vi "StopSong.vi"(8 "error in (no error)":errorcluster, 10 "Message Queues in":T1, 11 "UI Refs in":T2) -> (0 "error out":errorcluster, 2 "Message Queues out":T1, 3 "UI Refs out":T2)   [LabVIEW 2015]
uses:
  Controls & Type Defs/UI Data.ctl
  support/Message Queue/All Message Queues.ctl
  support/Message Queue/Message Cluster.ctl
  support/Message Queue/Enqueue Message (Single).vi
  support/Message Queue/Message Queue.lvlib
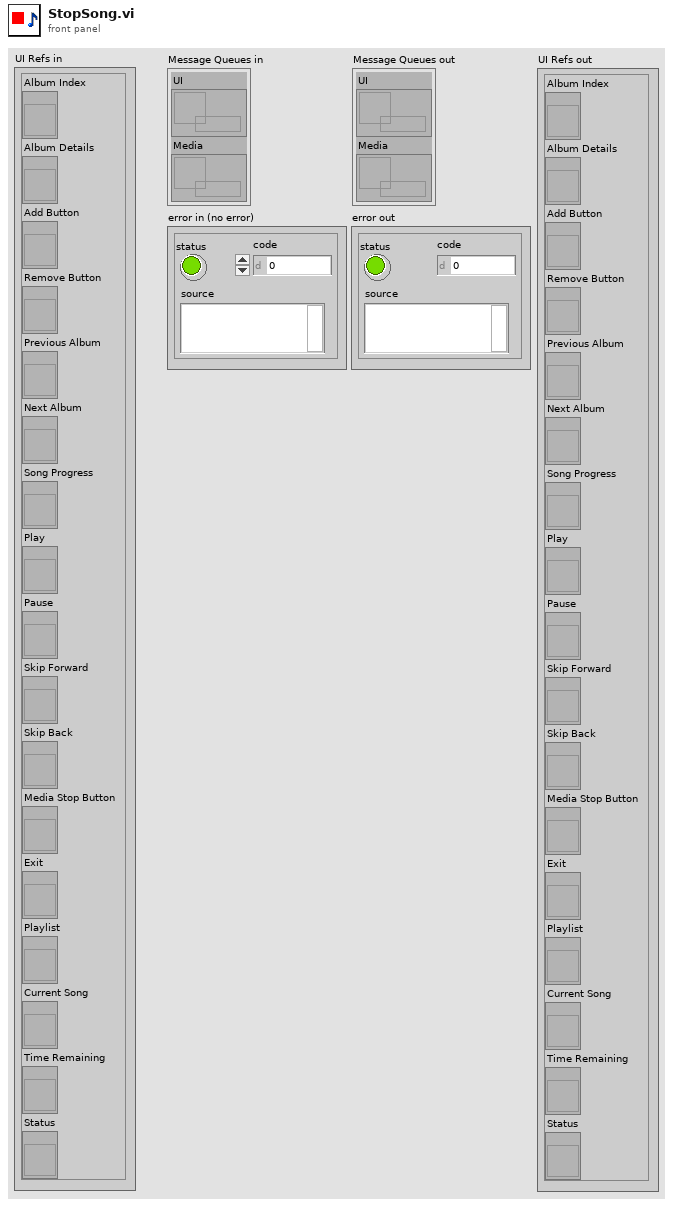
[diagram p1: front panel]
types:
  T1 = typedef "Message Queue.lvlib/All Message Queues.ctl" = cluster{"UI":refnum<queue>, "Media":refnum<queue>}
  T2 = typedef "UI Data.ctl" = cluster{"Album Index":refnum<vi>, "Album Details":refnum<vi>, "Add Button":refnum<vi>, "Remove Button":refnum<vi>, "Previous Album":refnum<vi>, "Next Album":refnum<vi>, "Song Progress":refnum<vi>, "Play":refnum<vi>, "Pause ":refnum<vi>, "Skip Forward":refnum<vi>, "Skip Back":refnum<vi>, "Media Stop Button":refnum<vi>, "Exit":refnum<vi>, "Playlist":refnum<vi>, "Current Song":refnum<vi>, "Time Remaining":refnum<vi>, "Status":refnum<vi>}
  T3 = enum8{"Enabled", "Disabled", "Disabled and Grayed Out"}
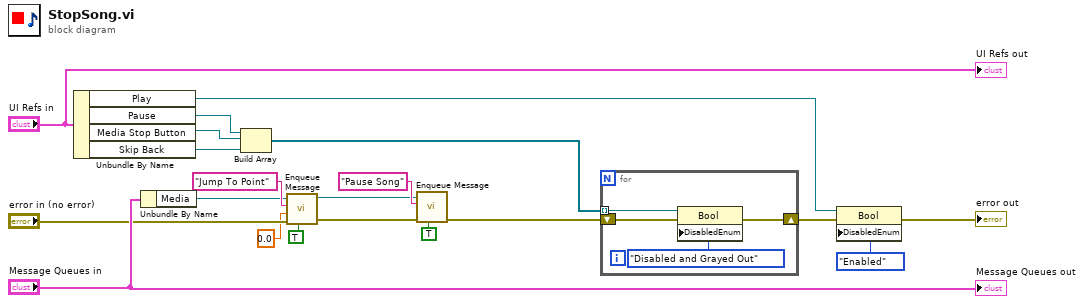
[diagram p0: block diagram]
diagram:
  n1 = Unbundle By Name("UI Refs in") -> ("Play"=w16:refnum<vi>, "Pause"=w18:refnum<vi>, "Media Stop Button"=w19:refnum<vi>, "Skip Back"=w20:refnum<vi>)
  n2 = Unbundle By Name("Message Queues in") -> ("Media"=w5:refnum<queue>)
  n3 = Build Array(w18, w19, w20) -> (w17:refnum<vi>[])
  n4 = call-poly "Enqueue Message.vi"("Priority Message? (F)"=TRUE, "error in (no error)"="error in (no error)", "Message Data"=0.0, "Message"="Jump To Point", "Message Queue"=w5) -> ("error out"=w7:errorcluster, "dup Message Queue"=w4:refnum<queue>)  [unwired: 5 in]
  n5 = call-poly "Enqueue Message.vi"("Priority Message? (F)"=TRUE, "error in (no error)"=w7, "Message"="Pause Song", "Message Queue"=w4) -> ("error out"=w6:errorcluster)  [unwired: 6 in, 1 out]
  n6 = for {
    shift-right: [w21] -> w14
    shift-left: w6 -> [w23]
    tunnel: w17 -> [w22] mode=indexing
    n7 = property class="Bool"(reference=w22, error in=w23, "DisabledEnum"=T3."Disabled and Grayed Out" ("Disabled")) -> (error out=w21:errorcluster)  [unwired: 1 out]
  }
  n8 = property class="Bool"(reference=w16, error in=w14, "DisabledEnum"=T3."Enabled" ("Disabled")) -> (error out=→"error out":errorcluster)  [unwired: 1 out]
  "UI Refs out" <- "UI Refs in"
  "Message Queues out" <- "Message Queues in"
